vi "Textframe Resize Policy to Enum.vi"(0 "Resize policy":T1) -> (2 "AutoSize":i32, 3 "WordWrap":i32)   [LabVIEW 2020, in "lvpptx.lvlib"]
uses:
  lvpptx.lvlib
  Textframe Resize Policy.ctl
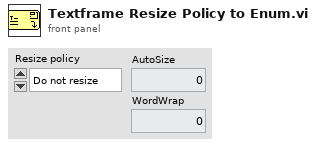
[diagram p1: front panel]
types:
  T1 = typedef "Textframe Resize Policy.ctl" = enum16{"Do not resize", "Expand horizontally", "Expand vertically"}
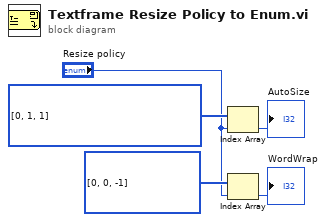
[diagram p0: block diagram]
diagram:
  w4 = i32[] [0, 0, -1] items=["msoTrue"=-1, "msoFalse"=0, "msoCTrue"=1, "msoTriStateToggle"=-3, "msoTriStateMixed"=-2] ("WordWrap")
  w5 = i32[] [0, 1, 1] items=["ppAutoSizeMixed"=-2, "ppAutoSizeNone"=0, "ppAutoSizeShapeToFitText"=1] ("AutoSize")
  n1 = Index Array(array=w5, index="Resize policy") -> (element=→"AutoSize":i32)
  n2 = Index Array(array=w4, index="Resize policy") -> (element=→"WordWrap":i32)
